vi "Server Loop.vi"(8 "error in (no error)":errorcluster, 11 "LabBOT in":refnum<class "LabBOT.lvclass">) -> (0 "error out":errorcluster)   [LabVIEW 2020, in "Rover.lvlib" / "LabBOT.lvclass"]
uses:
  LabBOT.lvclass
  LabBOT.lvclass/LabBOT.ctl
  <vilib>/MediaMongrels Ltd/WebSockets/Sockets/VISA TCP Listener/VISA TCP Listener.lvclass
  <vilib>/MediaMongrels Ltd/WebSockets/Sockets/Socket/Socket.lvclass
  <vilib>/MediaMongrels Ltd/WebSockets/WebSockets/WebSocket Server/WebSocket Server.lvclass
  Rover/Rover.lvclass
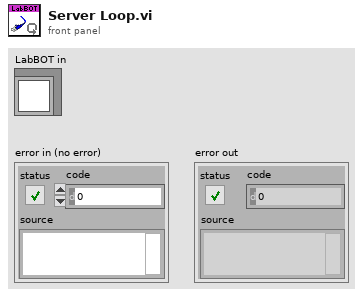
[diagram p1: front panel]
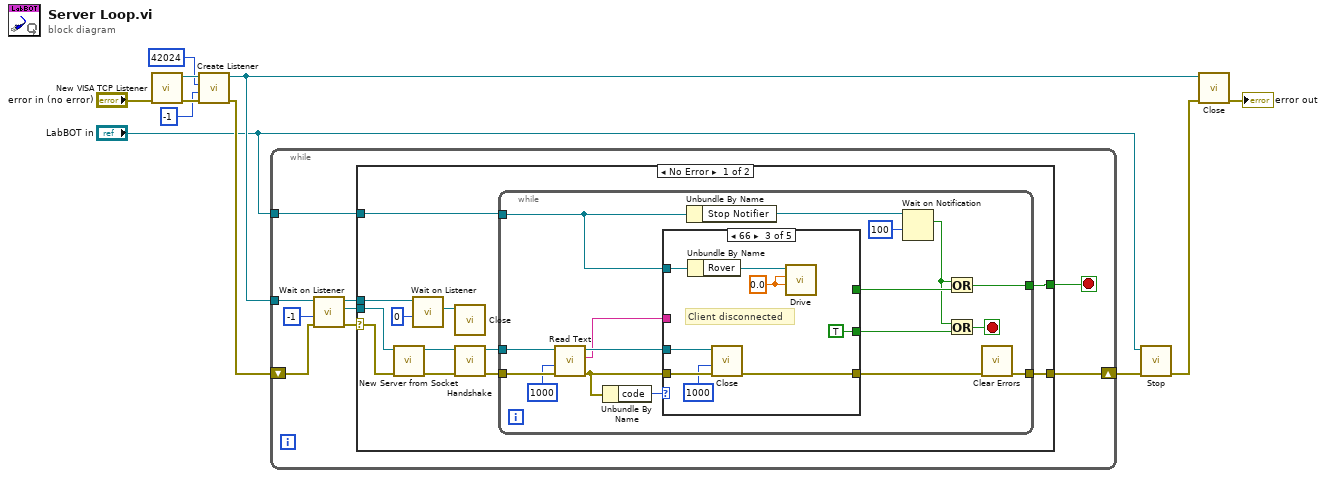
[diagram p0: block diagram]
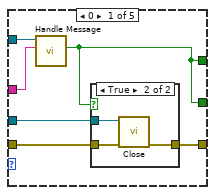
[diagram p2: hidden frame]
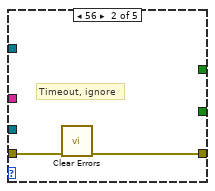
[diagram p4: hidden frame]
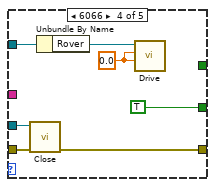
[diagram p5: hidden frame]
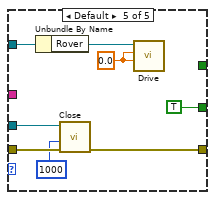
[diagram p6: hidden frame]
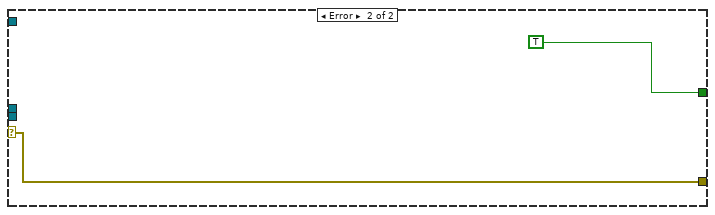
[diagram p7: hidden frame]
diagram:
  n1 = call <vilib>:"New VISA TCP Listener.vi"("error in (no error)"="error in (no error)") -> ("error out"=w10:errorcluster, "VISA TCP Listener out"=w11:refnum<class "VISA TCP Listener.lvclass">)  [unwired: 9 in]
  n2 = call-dynamic "Create Listener.vi"("error in (no error)"=w10, "timeout ms (5000)"=-1, "Port"=u16 42024, "VISA TCP Listener in"=w11) -> ("error out"=w6:errorcluster, "VISA TCP Listener out"=w5:refnum<class "VISA TCP Listener.lvclass">)  [unwired: 6 in]
  n3 = while {
    shift-right: [w15] -> w3
    shift-left: w6 -> [w13]
    tunnel: w5 -> [w14]
    tunnel: "LabBOT in" -> [w16]
    stop <- w17 stop-if-true
    n4 = call-dynamic "Wait on Listener.vi"("error in (no error)"=w13, "timeout ms (5000)"=-1, "VISA TCP Listener in"=w14) -> ("error out"=w20:errorcluster, "Socket out"=w19:refnum<class "Socket.lvclass">, "VISA TCP Listener out"=w18:refnum<class "VISA TCP Listener.lvclass">)  [unwired: 6 in]
    n5 = case shown="No Error" w20 {
      selector: w20 -> [w32 w85]
      tunnel: w19 -> [w31 _]
      tunnel: w18 -> [w23 _]
      tunnel: [w26 TRUE ("Close?")] -> w17
      tunnel: w16 -> [w25 _]
      tunnel: [w24 w85] -> w15
      frame No Error {
        n6 = call <vilib>:"New Server from Socket.vi"("error in (no error)"=w32, "Socket"=w31) -> ("error out"=w29:errorcluster, "WebSocket Server out"=w30:refnum<class "WebSocket Server.lvclass">)  [unwired: 8 in]
        n7 = call-dynamic "Wait on Listener.vi"("timeout ms (5000)"=0, "VISA TCP Listener in"=w23) -> ("Socket out"=w21:refnum<class "Socket.lvclass">)  [unwired: 7 in, 2 out]
        n8 = call-dynamic "Close.vi"("Socket in"=w21) -> ()  [unwired: 10 in, 1 out]
        n9 = call-dynamic "Handshake.vi"("error in (no error)"=w29, "WebSocket Connection in"=w30) -> ("error out"=w27:errorcluster, "WebSocket Connection out"=w28:refnum<class "WebSocket Server.lvclass">)  [unwired: 8 in]
        n10 = while {
          tunnel: w27 -> [w49]
          tunnel: [w34] -> w26
          tunnel: w28 -> [w48]
          tunnel: [w39] -> w24
          tunnel: w25 -> [w38]
          stop <- w35 stop-if-true
          n11 = call-dynamic "Read Text.vi"("error in (no error)"=w49, "timeout ms (5000)"=1000, "WebSocket in"=w48) -> ("error out"=w44:errorcluster, "Data"=w45:string, "WebSocket out"=w46:refnum<class "WebSocket Server.lvclass">)  [unwired: 6 in]
          n12 = Unbundle By Name(w44) -> ("code"=w47:i32)
          n13 = case shown="66" w47 {
            tunnel: w46 -> [w55 _ w65 w75 w82]
            tunnel: w45 -> [w53 _ _ _ _]
            tunnel: w44 -> [w54 w61 w66 w76 w83]
            tunnel: [w51 _ TRUE TRUE TRUE] -> w43
            tunnel: [w51 _ _ _ _] -> w42
            tunnel: w38 -> [w50 _ w68 w70 w77]
            tunnel: [w52 w60 w64 w73 w80] -> w40
            frame 0 {
              n14 = call "Handle Message.vi"("Message"=w53, "LabBOT in"=w50) -> ("Close?"=w51:bool)  [unwired: 8 in, 1 out]
              n15 = case shown="True" w51 {
                tunnel: w55 -> [_ w58]
                tunnel: w54 -> [w56 w59]
                tunnel: [w56 w57] -> w52
                frame False {
                }
                frame True {
                  n16 = call-dynamic "Close.vi"("error in (no error)"=w59, "WebSocket in"=w58) -> ("error out"=w57:errorcluster)  [unwired: 9 in]
                }
              }
            }
            frame 56 {
              # "Timeout, ignore"
              n17 = call <vilib>:"Clear Errors.vi"("error in (no error)"=w61) -> ("error out"=w60:errorcluster)  [unwired: 5 in, 1 out]
            }
            frame 66 {
              w67 = sgl 0.0 ("Drive")
              # "Client disconnected"
              n18 = Unbundle By Name(w68) -> ("Rover"=w62:refnum<class "Rover.lvclass">)
              n19 = call-dynamic "Close.vi"("error in (no error)"=w66, "timeout ms (5000)"=1000, "WebSocket in"=w65) -> ("error out"=w64:errorcluster)  [unwired: 8 in]
              n20 = call "Drive.vi"("Turn"=w67, "Drive"=w67, "Rover in"=w62) -> ()  [unwired: 7 in, 2 out]
            }
            frame 6066 {
              w72 = sgl 0.0 ("Drive")
              n21 = call-dynamic "Close.vi"("error in (no error)"=w76, "WebSocket in"=w75) -> ("error out"=w73:errorcluster)  [unwired: 9 in]
              n22 = Unbundle By Name(w70) -> ("Rover"=w71:refnum<class "Rover.lvclass">)
              n23 = call "Drive.vi"("Turn"=w72, "Drive"=w72, "Rover in"=w71) -> ()  [unwired: 7 in, 2 out]
            }
            frame Default {
              w79 = sgl 0.0 ("Drive")
              n24 = Unbundle By Name(w77) -> ("Rover"=w78:refnum<class "Rover.lvclass">)
              n25 = call-dynamic "Close.vi"("error in (no error)"=w83, "timeout ms (5000)"=1000, "WebSocket in"=w82) -> ("error out"=w80:errorcluster)  [unwired: 8 in]
              n26 = call "Drive.vi"("Turn"=w79, "Drive"=w79, "Rover in"=w78) -> ()  [unwired: 7 in, 2 out]
            }
          }
          n27 = Unbundle By Name(w38) -> ("Stop Notifier"=w37:refnum<notifier>)
          n28 = Wait on Notification(notifier=w37, timeout in ms (-1)=100) -> (notification=w33:bool)  [unwired: 2 in, 3 out]
          n29 = Or(x=w33, y=w42) -> (x .or. y?=w34:bool)
          n30 = Or(x=w33, y=w43) -> (x .or. y?=w35:bool)
          n31 = call <vilib>:"Clear Errors.vi"("error in (no error)"=w40) -> ("error out"=w39:errorcluster)  [unwired: 5 in, 1 out]
        }
      }
      frame Error {
      }
    }
  }
  n32 = call "Stop.vi"("error in (no error)"=w3, "LabBOT in"="LabBOT in") -> ("error out"=w2:errorcluster)  [unwired: 8 in, 1 out]
  n33 = call-dynamic "Close.vi"("error in (no error)"=w2, "VISA TCP Listener in"=w5) -> ("error out"=→"error out":errorcluster)  [unwired: 9 in]
